vi "Test Handler Default Formatter.vi"(8 "error in":errorcluster) -> (0 "error out":errorcluster)   [LabVIEW 2016, in "UT_Formatter.lvlib"]
doc: "Test the default formatter used by the handler when the Create Formatter function isn't called."
uses:
  UT_Formatter.lvlib
  Source/HSE-Logger/LogLevel.ctl
  Source/HSE-Logger/Handler/FileHandler/FileHandler.lvclass/FileHandler.ctl
  Source/HSE-Logger/Handler/FileHandler/FileHandler.lvclass
  <vilib>/addons/_JKI Toolkits/Caraya/classes/Test/Test.lvclass
  Source/HSE-Logger/hse-logger.lvlib
  Source/HSE-Logger/Formatter/Formatter.lvclass
  <vilib>/addons/_JKI Toolkits/Caraya/classes/Assert/Assert.lvclass
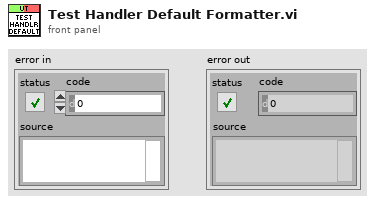
[diagram p1: front panel]
types:
  T1 = typedef "hse-logger.lvlib/LogLevel.ctl" = enum16{"DEBUG", "INFO", "WARNING", "ERROR", "CRITICAL"}
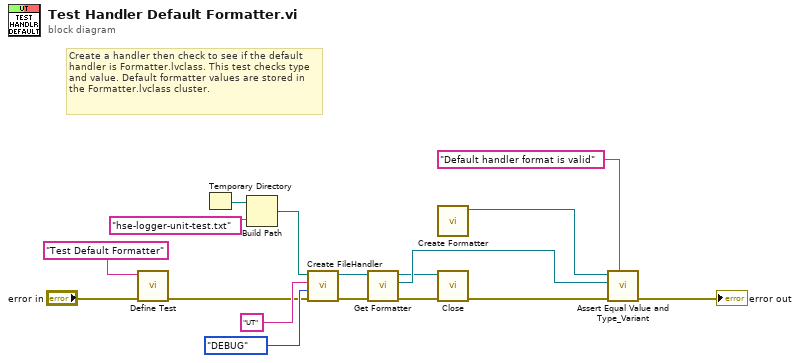
[diagram p0: block diagram]
diagram:
  # "Create a handler then check to see if the default handler is Formatter.lvclass. This test checks type and value. Default formatter values are stored in the Formatter.lvclass cluster."
  n1 = call <vilib>:"Define Test.vi"("error in (no error)"="error in", "Label (VI Title)"="Test Default Formatter") -> ("error out"=w9:errorcluster)  [unwired: 8 in, 1 out]
  n2 = Temporary Directory() -> (w3:path)
  n3 = Build Path(base path=w3, name or relative path="hse-logger-unit-test.txt") -> (appended path=w1:path)
  n4 = call "Create FileHandler.vi"("error in"=w9, "Level"=LogLevel."DEBUG", "Name"="UT", "Filepath"=w1) -> ("error out"=w8:errorcluster, "FileHandler out"=w7:refnum<class "FileHandler.lvclass">)  [unwired: 6 in]
  n5 = call "Get Formatter.vi"("error in"=w8, "FileHandler"=w7) -> ("error out"=w6:errorcluster, "Formatter"=w5:refnum<class "Formatter.lvclass">, "FileHandler out"=w4:refnum<class "FileHandler.lvclass">)  [unwired: 7 in]
  n6 = call "Create Formatter.vi"() -> ("Formatter out"=w13:refnum<class "Formatter.lvclass">)  [unwired: 10 in, 1 out]
  n7 = call-dynamic "Close.vi"("error in"=w6, "FileHandler in"=w4) -> ("error out"=w16:errorcluster)  [unwired: 8 in, 1 out]
  n8 = call <vilib>:"Assert Equal Value and Type_Variant.vi"("Label"="Default handler format is valid", "error in (no error)"=w16, "Y"=w5, "X"=w13) -> ("error out"=→"error out":errorcluster)  [unwired: 6 in, 1 out]
